vi "2014 Ball Detection.vi"() -> ()   [LabVIEW 2013]
uses:
  <vilib>/Rock Robotics/WPI/Camera/WPI_CameraSettings Read MJPG.ctl
  <vilib>/Rock Robotics/WPI/Camera/WPI_CameraImageSize.ctl
panel:
  out "Error":bool
  in  "Tabbed Info":T1(tab)
  in  "Annotations":enum16{"None", "Good", "All"}(ring)=enum."Good"
  out "Initial Mask":T2(plugin-control)
  out "Fitted Mask":T2(plugin-control)
  in  "Color Components":T3={"Hue"={243.23333311080933, 20.233333110809326}, "Sat"={125.60287475585938, 242.93045043945312}, "Val"={83.88507843017578, 225.38158416748047}} {"Val" scale=0.0..255.0; "Sat" scale=0.0..255.0; "Hue" scale=0.0..255.0 scale format="%#_3g"}
  in  "Camera IP":string="10.04.19.11"
  in  "Camera Settings":T4={"fps"=15, "compression"=5, "Image Size"=enum."320x240"}
  out "Bandwidth (Mbps)":dbl
  in  "Score Cutoff":dbl(slide)=70.58823529411765 scale=0.0..100.0
  in  "Area Size Limit %":dbl=0.4 format="%#_13g"
  in  "Targets":i32=3
  in  "Std Devs":cluster{"Hue":dbl, "Sat":dbl, "Val":dbl}={"Hue"=4.0, "Sat"=6.0, "Val"=4.0}
  out "Ranked Objects":T6(array[cluster]) {"Score" format="%#.1g"}
  out "Image":T2(plugin-control)
  # "Ranking Colors:\n1. green\n2. cyan\n3. magenta\n4. orange"
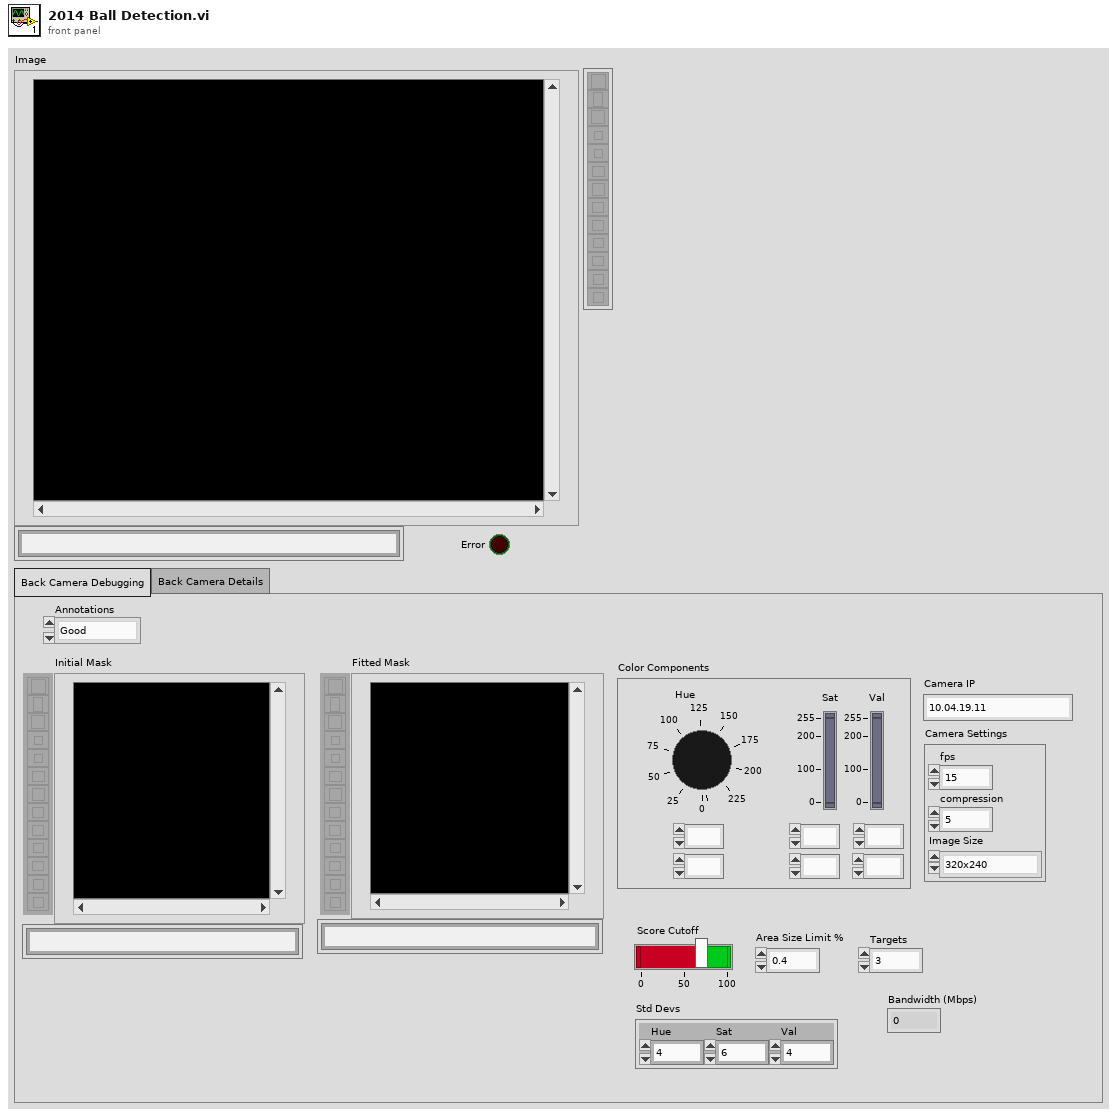
[diagram p1: front panel]
types:
  T1 = enum32{"Back Camera Debugging", "Back Camera Details"}
  T2 = typedef "IMAQ Image.ctl" = refnum<image>
  T3 = cluster{"Hue":cluster{dbl, dbl}, "Sat":cluster{dbl, dbl}, "Val":cluster{dbl, dbl}}
  T4 = typedef "WPI_CameraSettings Read MJPG.ctl" = cluster{"fps":i32, "compression":i32, "Image Size":T5}
  T5 = typedef "WPI_CameraImageSize.ctl" = enum16{"640x480", "320x240", "160x120"}
  T6 = cluster{"Score":sgl, "Fitted Circle":cluster{"Center":cluster{"X":sgl, "Y":sgl}, "Radius":dbl, "Circle Rect":cluster{"L":sgl, "T":sgl, "R":sgl, "B":sgl}, "Roundness":dbl, "SNR (dB)":dbl}, "Search Rect":cluster{"L":sgl, "T":sgl, "R":sgl, "B":sgl}, "Details":cluster{"Edge":sgl, "Area":sgl, "Circ":sgl, "Diam":sgl}}[]
  T7 = typedef "Image Type" = u32
  T8 = cluster{"Circle Found":bool, "Fitted Circle":cluster{"Center":cluster{"X":sgl, "Y":sgl}, "Radius":dbl, "Center":cluster{"X":sgl, "Y":sgl}, "Radius":dbl, "Roundness":dbl, "Strength":dbl, "SNR (dB)":dbl}, "Array":dbl[], "Sorted Data":dbl[][]}[]
  T9 = cluster{cluster{dbl, dbl}, cluster{dbl, dbl}, cluster{dbl, dbl}}
  T10 = cluster{"Score":dbl, "Fitted Circle":cluster{"Center (Pixels)":cluster{"X":sgl, "Y":sgl}, "Radius (Pixels)":dbl, "Circle Rect":cluster{"Left":sgl, "Top":sgl, "Right":sgl, "Bottom":sgl}, "Roundness (RW)":dbl, "Average SNR (dB)":dbl}, "Search Rect":cluster{"Left":sgl, "Top":sgl, "Right":sgl, "Bottom":sgl}, "Details":cluster{"Edges":sgl, "Circ/Rect":sgl, "Diam/Diam":sgl, "Circularity":sgl}}[]
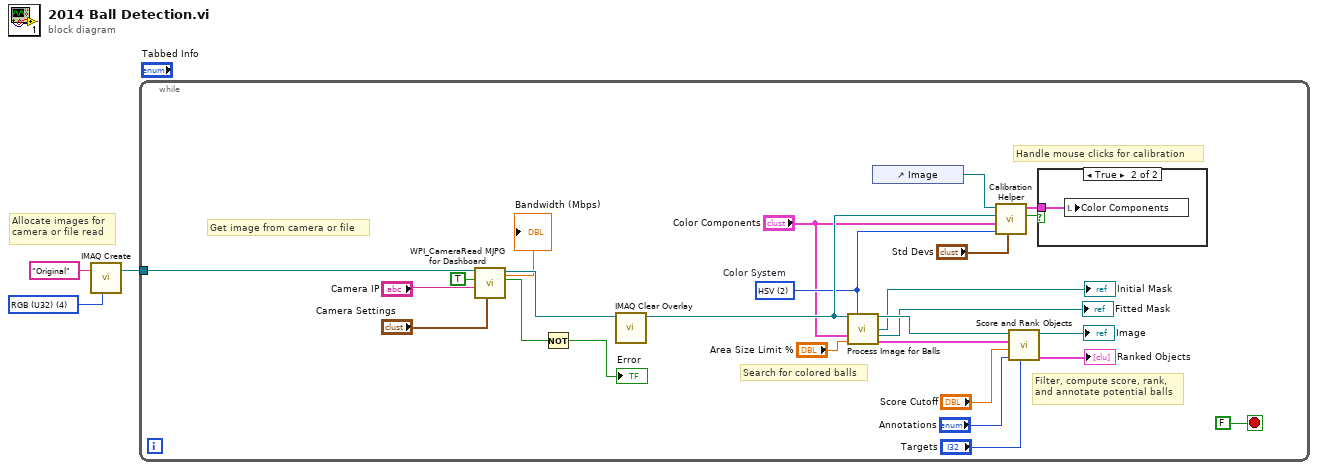
[diagram p0: block diagram]
diagram:
  w3 = T7 4 items=["Grayscale (U8)", "Grayscale (I16)", "Grayscale (SGL)", "Complex (CSG)", "RGB (U32)", "HSL (U32)", "RGB (U64)", "Grayscale (U16)"] ("Image Type")
  # "Allocate images for\ncamera or file read"
  n1 = call "IMAQ Create"("Image Name"="Original", "Image Type"=w3) -> ("New Image"=w1:T2)  [unwired: 3 in, 1 out]
  n2 = while {
    tunnel: w1 -> [w27]
    stop <- FALSE stop-if-true
    w14 = u16 2 items=["RGB", "HSL", "HSV", "HSI"]  # Color System
    # "Handle mouse clicks for calibration"
    # "Search for colored balls"
    # "Filter, compute score, rank,\nand annotate potential balls"
    # "Get image from camera or file"
    n3 = call <vilib>:"WPI_CameraRead MJPG for Dashboard.vi"("Camera Settings"="Camera Settings", "Camera IP"="Camera IP", "Enable"=TRUE, "Refnum in"=w27) -> ("Active"=w6:bool, "Refnum out"=w29:T2, "Bandwidth (Mbps)"=→"Bandwidth (Mbps)":dbl)  [unwired: 4 in, 1 out]
    n4 = Not(x=w6) -> (.not. x?=→"Error":bool)
    n5 = call "IMAQ Clear Overlay"("Image"=w29) -> ("Image Out"=w21:T2)  [unwired: 9 in, 1 out]
    n6 = call "Process Image for Balls.vi"("Src Image"=w21, "Color Mode 2"=w14, "Color"="Color Components", "Area Cutoff %"="Area Size Limit %") -> ("Src Image Out"=w19:T2, "First Threshold"=→"Initial Mask":T2, "Fitted"=→"Fitted Mask":T2, "Potential"=w18:T8)  [unwired: 8 in]
    n7 = control-ref of="Image"() -> (w13:refnum<vi>)
    n8 = call "Calibration Helper.vi"("Std Devs"="Std Devs", "Color Mode"=w14, "Color Components"="Color Components", "Image"=w21, "Image Ctl Refnum"=w13) -> ("Changed"=w10:bool, "output color"=w12:T9)  [unwired: 5 in]
    n9 = call "Score and Rank Objects.vi"("Targets"="Targets", "Annotations"="Annotations", "Score Limit"="Score Cutoff", "Object Info"=w18, "Image in"=w19) -> ("Object Info"=→"Ranked Objects":T10, "Annotated Image"=→"Image":T2)  [unwired: 5 in]
    n10 = case shown="True" w10 {
      tunnel: w12 -> [_ w30]
      frame False {
      }
      frame True {
        n11 = local write "Color Components"(w30) -> ()
      }
    }
  }
